vi "ThreadCfg - Control Dialog UI.vi"(7 "rxPacket?":bool, 9 "threadManagement":T2, 10 "threadPeriodRef":T3=enum."Async") -> (0 "priorityState":T1(ring), 1 "pclDecimationState":T1(ring), 2 "loopPeriodState":T1(ring))   [LabVIEW 2016, in "UDP-Custom-Device System Explorer.lvlib"]
uses:
  UDP-Custom-Device System Explorer.lvlib
  Types/Threading/Thread Sync Reference.ctl
  Types/Threading/Thread Management.ctl
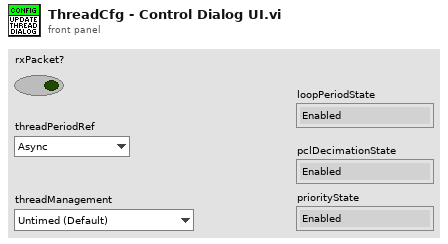
[diagram p1: front panel]
types:
  T1 = enum8{"Enabled", "Disabled", "Disabled and Grayed Out"}
  T2 = typedef "UDP-Custom-Device System Explorer.lvlib/Thread Management.ctl" = enum16{"Untimed (Default)", "Timed (High Priority)"}
  T3 = typedef "UDP-Custom-Device System Explorer.lvlib/Thread Sync Reference.ctl" = enum16{"PCL", "Async"}
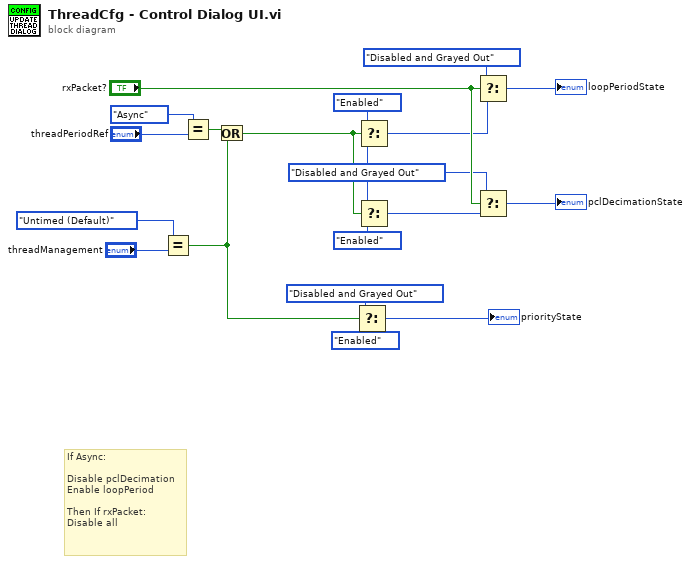
[diagram p0: block diagram]
diagram:
  w9 = T1."Disabled and Grayed Out" ("Disabled")
  # "If Async:\n\nDisable pclDecimation\nEnable loopPeriod\n\nThen If rxPacket:\nDisable all"
  n1 = Equal?(x=Thread_Management."Untimed (Default)", y="threadManagement") -> (x = y?=w1:bool)
  n2 = Equal?(x=Thread_Sync_Reference."Async", y="threadPeriodRef") -> (x = y?=w6:bool)
  n3 = Or(x=w6, y=w1) -> (x .or. y?=w5:bool)
  n4 = Select(t=T1."Disabled and Grayed Out" ("Disabled"), s=w1, f=T1."Enabled" ("Disabled")) -> (s? t:f=→"priorityState":T1)
  n5 = Select(t=T1."Enabled" ("Disabled"), s=w5, f=w9) -> (s? t:f=w10:T1)
  n6 = Select(t=w9, s=w5, f=T1."Enabled" ("Disabled")) -> (s? t:f=w11:T1)
  n7 = Select(t=T1."Disabled and Grayed Out" ("Disabled"), s="rxPacket?", f=w10) -> (s? t:f=→"loopPeriodState":T1)
  n8 = Select(t=w9, s="rxPacket?", f=w11) -> (s? t:f=→"pclDecimationState":T1)
